vi "Untitled 1.vi"() -> ()   [LabVIEW 2020]
panel:
  in  "Numeric":dbl
  out "sub":dbl(slide) scale=0.0..100.0
  out "sum":dbl
  in  "y":dbl=66.0
  in  "x":dbl
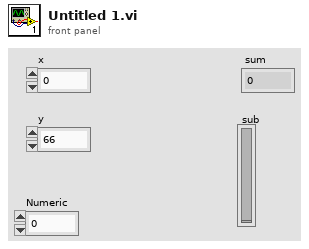
[diagram p1: front panel]
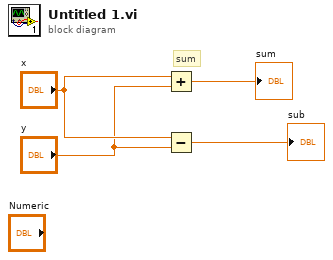
[diagram p0: block diagram]
diagram:
  # "sum"
  n1 = Add(x="x", y="y") -> (x+y=→"sum":dbl)
  n2 = Subtract(x="x", y="y") -> (x-y=→"sub":dbl)
